vi "deviceAnalysisTest_DigitalTach.vi"() -> ()   [LabVIEW 2017]
uses:
  <vilib>/addons/InsightCM/MessageBus/Base/KeyValuePairs.ctl
  <vilib>/addons/InsightCM/MessageBus/Base/controls/AlarmRuleEntry.ctl
  <vilib>/addons/InsightCM/Devices/Shared/DataAccessors/controls/channelType_StatusLookup.ctl
  <vilib>/addons/InsightCM/MessageBus/Base/ConfigurableMetric.ctl
  <vilib>/addons/InsightCM/Utilities/ChannelStatus/controls/status.ctl
  <vilib>/addons/InsightCM/Utilities/ChannelStatus/controls/statusState.ctl
  <vilib>/addons/InsightCM/Devices/Shared/ConfigurationParsing/controls/filePaths.ctl
panel:
  out "seconds":i32
  out "logical OR":bool
  in  "Tachometer":cluster{"RPM":sgl}={"RPM"=60.0} {"RPM" scale=1.0..6000.0}
  in  "milliseconds to wait":u32=100
  in  "Tab Control":T1(tab)
  in  "Root Directory":path=path "C:/Users/Administrator/Desktop/testDevice files/speedProfile"
  in  "Configuration Files":T2={"AlarmRules"=path "AlarmRules.json", "MetricCfg"=path "MetricConfigs.json", "HierarchyNode"=path "Hierarchy.json", "DeviceModel"=path "DeviceModel.json"}
  in  "sampling info":cluster{"Fs":dbl, "#s":dbl}={"Fs"=10000.0, "#s"=10000.0} {"Fs" format="%.2p"}
  in  "Vibration":T3(array[cluster])
  out "Waveform Graph":waveform(dbl)[](graph)
  out "Waveform Graph 2":waveform(sgl)[](graph)
  out "FeatureLookup":variant
  in  "stop":bool
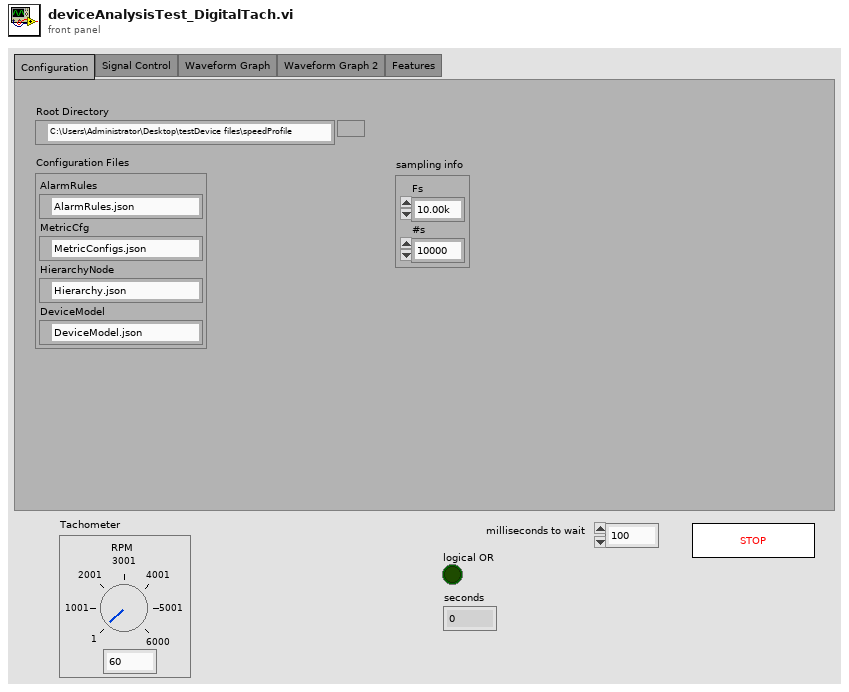
[diagram p1: front panel]
types:
  T1 = enum32{"Configuration", "Signal Control", "Waveform Graph", "Waveform Graph 2", "Features"}
  T2 = typedef "ConfigurationParsing.lvlib/filePaths.ctl" = cluster{"AlarmRules":path, "MetricCfg":path, "HierarchyNode":path, "DeviceModel":path}
  T3 = cluster{"order.":dbl, "mag (rms)":dbl, "phase (°)":dbl}[][]
  T4 = typedef "ChannelStatus.lvlib/statusState.ctl" = cluster{"channelAlias":string, "current":T5, "previous":T5, "changed":bool}
  T5 = typedef "ChannelStatus.lvlib/status.ctl" = enum16{"init", "ok", "open", "short", "outOfRange"}
  T6 = typedef "ConfigurableMetric.ctl" = cluster{"Id":i32, "MetricType":string, "Name":string, "Locked":bool, "Properties":T7}
  T7 = typedef "KeyValuePairs.ctl" = cluster{"Key":string, "Value":string}[]
  T8 = cluster{"order.":dbl, "mag (rms)":dbl, "phase (°)":dbl}[]
  T9 = typedef "AlarmRuleEntry.ctl" = cluster{"Id":i32, "State":string, "Path":string, "Message":string, "DeviceOnly":bool, "Configuration":cluster{"Condition":string, "SetPoint":string, "Type":string, "Hysteresis":dbl, "OnDelaySeconds":dbl, "OffDelaySeconds":dbl}, "Severity":i32}
  T10 = typedef "ConfigurationParsing.lvlib/DeviceConfigData.ctl" = cluster{"Device Info":T11, "AcquisitionProperties":variant, "Channels":variant[], "StreamingProperties":variant, "DeviceSystemProperties":variant}
  T11 = typedef "ConfigurationParsing.lvlib/deviceInfo.ctl" = cluster{"Config Version":string, "DeviceID":string}
  T12 = typedef "DeviceModel.ctl" = cluster{"AssetModel":T13, "SoftwareModel":T14}
  T13 = typedef "AssetModel.ctl" = cluster{"Id":i32, "PhysicalName":string, "LogicalName":string, "PluginCodename":string, "FirmwareInfo":string, "HardwareConfig":string, "SoftwareConfigId":i32, "HierarchyNodeId":i32}
  T14 = typedef "SoftwareModel.ctl" = cluster{"Id":i32, "DeviceAssetModelId":i32, "Version":string, "Config":string, "DeviceProperties":T7, "Channels":T15[]}
  T15 = typedef "BlueRidgeChannel.ctl" = cluster{"Id":i32, "ChannelId":string, "Name":string, "ChannelCategory":string, "ChannelType":string, "ChannelTypeList":string, "HierarchyNodeId":i32, "Enabled":bool, "Properties":T7, "MetricConfigurations":T16[]}
  T16 = typedef "MetricConfiguration.ctl" = cluster{"Id":i32, "ChannelCategory":string, "MeasurementType":string, "Metrics":T17[]}
  T17 = typedef "MetricInstance.ctl" = cluster{"Id":i32, "Codename":string, "DisplayName":string, "Unit":string, "Unscaled":bool, "Locked":bool, "TagPath":string, "Properties":T7}
  T18 = cluster{"AlarmRules":variant, "MetricCfg":variant, "HierarchyNode":variant, "DeviceConfig":T10, "DeviceModel":T12}
  T19 = typedef "AnalysisDevice.ctl" = cluster{"Device Id":string, "Dynamic Channels":T20[], "Static Channels":T28[]}
  T20 = typedef "AnalysisDynamicChannel.ctl" = cluster{"ChannelName":string, "Sensor Type":T21, "Conversion Op":T22, "Features":T23[], "Data":waveform(sgl), "Speed":sgl, "SP Index":i32, "Properties":variant, "Data Valid":bool, "Calc Measurement Type":T27}
  T21 = typedef "AnalysisSensorType.ctl" = enum16{"Accelerometer", "Velocity", "Displacement", "Tachometer", "Tempertature ", "dynamicVoltage", "Voltage", "Current", "Microphone", "Resistance", "Digital Input", "<Unknown>"}
  T22 = typedef "AnalysisConversionOp.ctl" = enum16{"none", "singleInt", "doubleInt", "singleDiff", "doubleDiff"}
  T23 = typedef "AnalysisFeature.ctl" = cluster{"Type":i32, "Code Name":string, "Unit":string, "Display Name":string, "Value":sgl, "Start":dbl, "Stop":dbl, "Band Domain":T24, "Band Calc":T25, "Amplitude Scale":T26, "Tag Path":string, "Conversion Op (phase sb only)":T22, "sbp code letter":string}
  T24 = typedef "AnalysisBandDomain.ctl" = enum16{"Frequency", "CPM", "Orders"}
  T25 = typedef "AnalysisBandCalculation.ctl" = enum16{"Total", "Max", "Phase"}
  T26 = typedef "AnalysisBandAmplitudeScale.ctl" = enum16{"rms", "peak", "pk-pk", "phase", "<none>"}
  T27 = typedef "AnalysisCalculatedMeasurementType.ctl" = enum16{"acceleration", "velocity", "displacement", "tachometer", "speed", "temperature", "voltage", "current", "resistance", "digitalInput", "<Unknown>"}
  T28 = typedef "AnalysisStaticChannel.ctl" = cluster{"ChannelName":string, "Sensor Type":T21, "Features":T23[], "Properties":variant, "Data Valid":bool, "Calc Measurement Type":T27, "Acquisition Timestamp":timestamp}
  T29 = typedef "AnalysisState.ctl" = cluster{"Properties":cluster{"File Properties":variant, "Static Properties":variant, "Waveform Properties":variant}, "Properties Initialized?":bool, "Device":T19, "Speed Profiles":T30[]}
  T30 = typedef "AnalysisSpeedProfile.ctl" = cluster{"t0":dbl, "pulse positions":sgl[], "speed":dbl}
  T31 = typedef "AnalysisBOP.lvlib/AnalysisGroups.ctl" = cluster{"StaticChannels":T32[], "TachVibrationGroups":T34[]}
  T32 = typedef "AnalysisBOP.lvlib/GeneralStaticChanAnalysisCfg.ctl" = cluster{"Wfm Index":i32, "ChannelName":string, "ChannelID":string, "bounds":T33, "TagPath":string, "Triggerable":bool}
  T33 = typedef "ChannelStatus.lvlib/outOfRangeBounds.ctl" = cluster{"maximum":dbl, "minimum":dbl}
  T34 = typedef "AnalysisBOP.lvlib/TachVibrationGroupCfg.ctl" = cluster{"TachometerChanAnalysisConfig":T35, "AnalysisChannels":T36[]}
  T35 = typedef "AnalysisBOP.lvlib/TachometerChanAnalysisCfg.ctl" = cluster{"Wfm Index":i32, "ChannelName":string, "ChannelID":string, "PulsesPerRevolution":sgl, "TachometerThreshold":sgl, "TachometerSlope":string, "TachometerHysteresis":sgl, "sampleRate":dbl, "tachometerType":string, "Analysis Wfm Index":i32}
  T36 = typedef "AnalysisBOP.lvlib/VibrationChanAnalysisCfg.ctl" = cluster{"Wfm Index":i32, "ChannelName":string, "ChannelID":string, "speedRatio":dbl, "MeasurementType":string}
  T37 = typedef "channelType_StatusLookup.ctl" = enum16{"Static", "Dynamic"}
  T38 = typedef "rolloverState.ctl" = cluster{"prev value":u32, "total add":dbl}
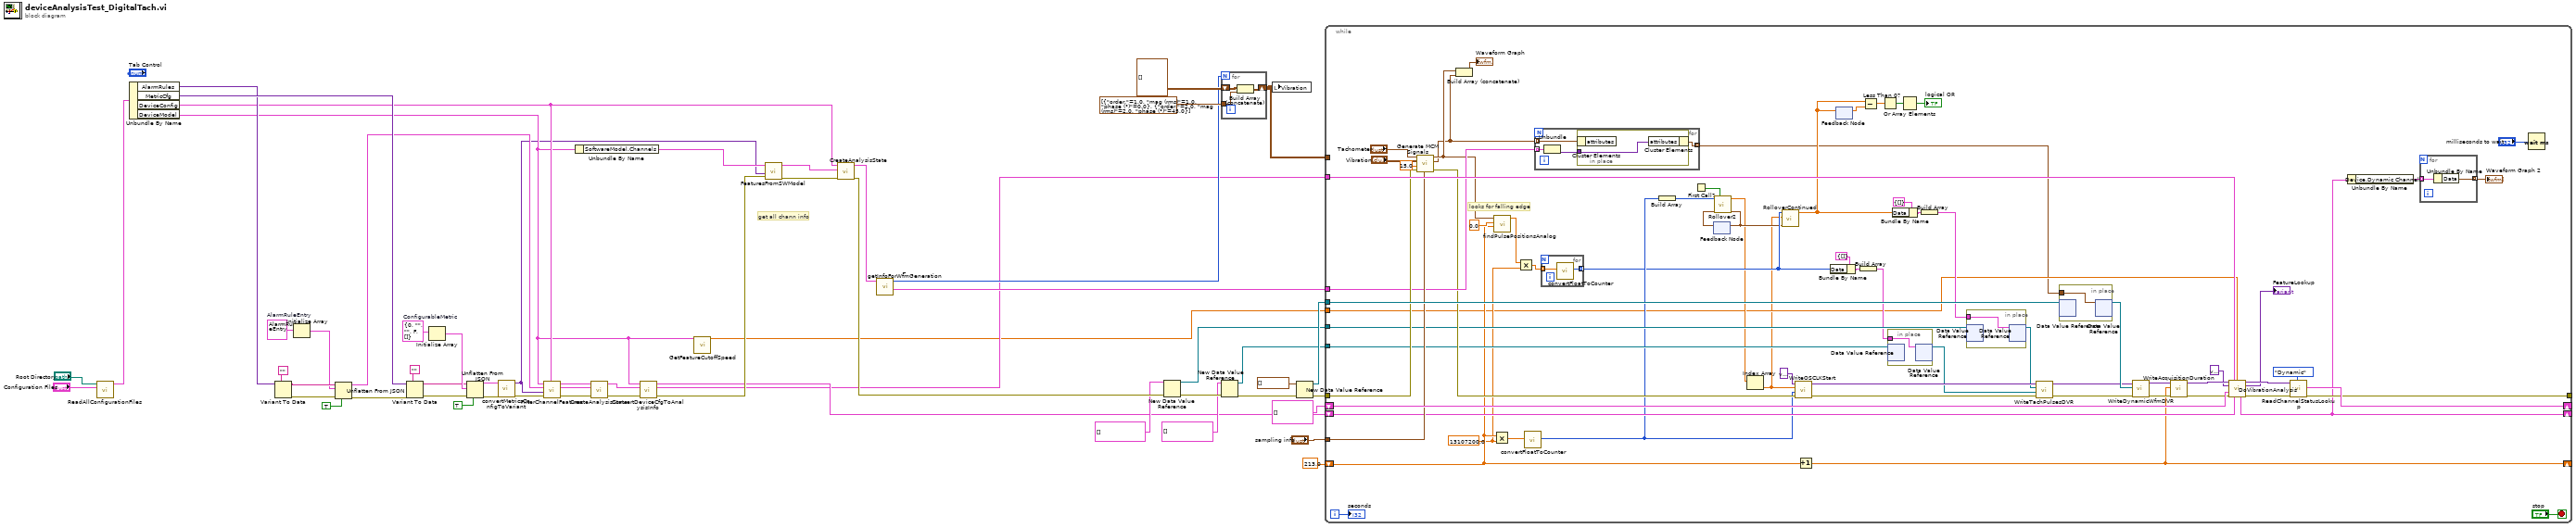
[diagram p0: block diagram]
diagram:
  w12 = T6 {"Id"=0, "MetricType"="", "Name"="", "Locked"=FALSE, "Properties"=[]}  # ConfigurableMetric
  w40 = T9 {"Id"=0, "State"="", "Path"="", "Message"="", "DeviceOnly"=FALSE, "Configuration"={"Condition"="", "SetPoint"="", "Type"="", "Hysteresis"=0.0, "OnDelaySeconds"=0.0, "OffDelaySeconds"=0.0}, "Severity"=0}  # AlarmRuleEntry
  # "get all chann info"
  n1 = call <vilib>:"ReadAllConfigurationFiles.vi"("Configuration Files"="Configuration Files", "Root Directory"="Root Directory") -> ("Configuration"=w52:T18)  [unwired: 6 in, 3 out]
  n2 = Unbundle By Name(w52) -> ("AlarmRules"=w37:variant, "MetricCfg"=w46:variant, "DeviceConfig"=w22:T10, "DeviceModel"=w5:T12)
  n3 = Variant To Data(type="", Variant=w37) -> (data=w41:string, error out=w43:errorcluster)  [unwired: 1 in]
  n4 = Initialize Array(w40) -> (w39:T9[])  [unwired: 1 in]
  n5 = Unflatten From JSON(JSON string=w41, type and defaults=w39, default null elements? (F)=TRUE, error in (no error)=w43) -> (value=w23:T9[], error out=w38:errorcluster)  [unwired: 3 in]
  n6 = Variant To Data(error in=w38, type="", Variant=w46) -> (data=w47:string, error out=w50:errorcluster)
  n7 = Initialize Array(w12) -> (w48:T6[])  [unwired: 1 in]
  n8 = Unflatten From JSON(JSON string=w47, type and defaults=w48, default null elements? (F)=TRUE, error in (no error)=w50) -> (value=w45:T6[], error out=w36:errorcluster)  [unwired: 3 in]
  n9 = call <vilib>:"convertMetricsConfigToVariant.vi"("error in (no error)"=w36, "MetricInstanceConfigs"=w45) -> ("error out"=w53:errorcluster, "metricInstanceConfig"=w1:variant)  [unwired: 8 in]
  n10 = call <vilib>:"FilterChannelFeatures.vi"("DeviceConfig"=w22, "error in (no error)"=w53, "Metric Lookup"=w1, "AlarmRules"=w23, "DeviceModel"=w5) -> ("error out"=w56:errorcluster, "Device"=w54:T19, "DeviceConfig Out"=w55:T10)  [unwired: 3 in, 1 out]
  n11 = Unbundle By Name(w5) -> ("SoftwareModel.Channels"=w13:T15[])
  n12 = call <vilib>:"CreateAnalysisState.vi"("error in (no error)"=w56, "Device"=w54, "DeviceConfig"=w55) -> ("error out"=w11:errorcluster, "Analysis State"=w10:T29)  [unwired: 7 in]
  n13 = call <vilib>:"ConvertDeviceCfgToAnalysisInfo.vi"("error in (no error)"=w11, "Analysis State"=w10, "DeviceModel"=w5) -> ("error out"=w9:errorcluster, "AnalysisGroups"=w7:T31, "Analysis State out"=w8:T29)  [unwired: 5 in, 1 out]
  n14 = call <vilib>:"GetFeatureCutoffSpeed.vi"("DeviceModel"=w5) -> ("featureCutoffSpeed"=w4:dbl)  [unwired: 10 in]
  n15 = call <vilib>:"FeaturesFromSWModel.vi"("error in (no error)"=w9, "Band Cache"=w1, "Channels"=w13) -> ("error out"=w3:errorcluster, "Device"=w2:T19)  [unwired: 7 in]
  n16 = call <vilib>:"CreateAnalysisState.vi"("error in (no error)"=w3, "Device"=w2, "DeviceConfig"=w22) -> ("error out"=w19:errorcluster, "Analysis State"=w24:T29)  [unwired: 7 in]
  n17 = call <vilib>:"_getInfoForWfmGeneration.vi"("Analysis State"=w24) -> ("wfm info"=w25:cluster{i32, "variant":variant}[], "number of channels"=w26:i32)  [unwired: 9 in]
  n18 = New Data Value Reference(data value=cluster{"Data":dbl[]}[] [] ("Keyphasor Pulses"), error in=w19) -> (data value reference=w15:refnum<data-value>, error out=w20:errorcluster)
  n19 = New Data Value Reference(data value=cluster{"Data":u32[]}[] [] ("Keyphasor Pulses U32"), error in=w20) -> (data value reference=w16:refnum<data-value>, error out=w21:errorcluster)
  n20 = for {
    N: w26 -> [_]
    tunnel: T8 [{"order."=1.0, "mag (rms)"=1.0, "phase (°)"=0.0}, {"order."=2.0, "mag (rms)"=2.0, "phase (°)"=45.0}] ("Vibration") -> [w59]
    shift-right: [w58] -> w28
    shift-left: T3 [] -> [w57]
    n21 = Build Array (concatenate)(w57, w59) -> (w58:T3)
  }
  n22 = local write "Vibration"(w28) -> ()
  n23 = New Data Value Reference(data value=waveform(sgl)[] [] ("wfmData"), error in=w21) -> (data value reference=w32:refnum<data-value>, error out=w33:errorcluster)
  n24 = while {
    tunnel: w33 -> [w117]
    tunnel: w7 -> [w128]
    shift-right: [w127] -> _
    shift-left: T4[] [] ("channel status") -> [w126]
    tunnel: w32 -> [w121]
    tunnel: "sampling info" -> [w115]
    tunnel: w28 -> [_]
    tunnel: [w109] -> _
    tunnel: w25 -> [w108]
    shift-right: [w106] -> _
    shift-left: w8 -> [w107]
    tunnel: w16 -> [w96]
    tunnel: w15 -> [w97]
    shift-right: [w88] -> _
    shift-left: 213.0 -> [w87]
    tunnel: w4 -> [w72]
    i -> [w66]
    stop <- "stop" stop-if-true
    w85 = 13107200.0
    # "looks for falling edge"
    n25 = call <vilib>:"Generate MCM Signals.vi"("sampling info"=w115, "error in"=w117, "square wave duty cycle (%)"=15.0, "Vibration"="Vibration", "Tachometer"="Tachometer") -> ("error out"=w98:errorcluster, "Vibration signals"=w62:waveform(dbl)[], "Tach signal"=w63:waveform(dbl))  [unwired: 4 in]
    n26 = Build Array (concatenate)(w63, w62) -> (→"Waveform Graph":waveform(dbl)[])
    n27 = Multiply(x=w87, y=w85) -> (x*y=w80:dbl)
    n28 = call <vilib>:"findPulsePositionsAnalog.vi"("t0"=w87, "Level"=0.0, "Tach signal"=w63) -> ("pulse positions"=w86:dbl[])  [unwired: 8 in]
    n29 = Multiply(x=w86, y=w85) -> (x*y=w81:dbl[])
    n30 = call <vilib>:"convertFloatToCounter.vi"("Numeric"=w80) -> ("Counter Version"=w78:u32)  [unwired: 10 in]
    n31 = for {
      tunnel: w62 -> [w137] mode=indexing
      tunnel: w108 -> [w138] mode=indexing
      tunnel: [w136] -> w65 mode=indexing
      n32 = Unbundle(w138) -> ("variant"=w135:variant)  [unwired: 1 out]
      n33 = in-place {
        in-place-border: w135 -> [w139]
        n34 = in-place-cluster #1(w137) -> ()  [unwired: 1 out]
        n35 = in-place-cluster #1("attributes"=w139) -> (w136:waveform(dbl))
      }
    }
    n36 = for {
      tunnel: w81 -> [w130] mode=indexing
      tunnel: [w129] -> w75 mode=indexing
      n37 = call <vilib>:"convertFloatToCounter.vi"("Numeric"=w130) -> ("Counter Version"=w129:u32)  [unwired: 10 in]
    }
    n38 = Build Array(w78) -> (w76:u32[])
    n39 = First Call?() -> (First Call?: T/F=w79:bool)
    n40 = feedback #2() -> (w77:T38)  [unwired: 1 in]
    n41 = call <vilib>:"Rollover2.vi"("reset"=w79, "rollover state"=w77, "counter"=w76) -> ("rollover state"=w74:T38, "counter"=w73:dbl[])  [unwired: 7 in]
    n42 = feedback-in #2(w74) -> ()
    n43 = Index Array(array=w73) -> (element=w60:dbl)  [unwired: 1 in]
    n44 = call <vilib>:"RolloverContinued.vi"("rollover state"=w74, "OSClkStart"=w60, "counter"=w75) -> ("this block"=w71:dbl[])  [unwired: 5 in, 3 out]
    n45 = call <vilib>:"WriteOSCLKStart.vi"("error in (no error)"=w98, "osclkStart U32"=w78, "osclkStart"=w60, "variant"=variant) -> ("error out"=w101:errorcluster, "variant"=w102:variant)  [unwired: 6 in]
    n46 = Increment(x=w87) -> (x+1=w88:dbl)
    n47 = Bundle By Name(cluster=cluster{"Data":u32[]} {"Data"=[]} ("PulsePositions"), "Data"=w75) -> (w84:cluster{"Data":u32[]})
    n48 = feedback-in #3(w71) -> ()
    n49 = feedback #3() -> (w70:dbl[])  [unwired: 1 in]
    n50 = Build Array(w84) -> (w82:cluster{"Data":u32[]}[])
    n51 = Subtract(x=w71, y=w70) -> (x-y=w69:dbl[])
    n52 = Less Than 0?(x=w69) -> (x < 0?=w68:bool[])
    n53 = in-place {
      in-place-border: w82 -> [w131]
      n54 = in-place-dvr #4(w96) -> ()  [unwired: 2 out]
      n55 = in-place-dvr #4(w131) -> (w95:refnum<data-value>)  [unwired: 1 out]
    }
    n56 = Bundle By Name(cluster=cluster{"Data":dbl[]} {"Data"=[]} ("PulsePositions"), "Data"=w71) -> (w90:cluster{"Data":dbl[]})
    n57 = Or Array Elements(Boolean array=w68) -> (logical OR=→"logical OR":bool)
    n58 = Build Array(w90) -> (w89:cluster{"Data":dbl[]}[])
    n59 = in-place {
      in-place-border: w89 -> [w132]
      n60 = in-place-dvr #5(w97) -> ()  [unwired: 2 out]
      n61 = in-place-dvr #5(w132) -> (w94:refnum<data-value>)  [unwired: 1 out]
    }
    n62 = call <vilib>:"WriteTachPulsesDVR.vi"("error in (no error)"=w101, "tachometer pulses U32"=w95, "tachometerPulsesDVR"=w94, "variant"=w102) -> ("error out"=w100:errorcluster, "variant"=w93:variant)  [unwired: 6 in]
    n63 = in-place {
      in-place-border: w65 -> [w140]
      n64 = in-place-dvr #6(w121) -> ()  [unwired: 2 out]
      n65 = in-place-dvr #6(w140) -> (w120:refnum<data-value>)  [unwired: 1 out]
    }
    n66 = call <vilib>:"WriteDynamicWfmDVR.vi"("error in (no error)"=w100, "dynamic Wfm DVR"=w120, "variant"=w93) -> ("error out"=w125:errorcluster, "variant"=w124:variant)  [unwired: 7 in]
    n67 = call <vilib>:"WriteAcquisitionDuration.vi"("error in (no error)"=w125, "acquisitionDuration"=w88, "variant"=w124) -> ("error out"=w122:errorcluster, "variant"=w123:variant)  [unwired: 7 in]
    n68 = call <vilib>:"DoVibrationAnalysis.vi"("variant"=w123, "AnalysisGroups"=w128, "FeatureSpeedCutoff"=w72, "featureLookup"=variant, "channel status"=w126, "error in (no error)"=w122, "Analysis State"=w107) -> ("variant out"=w112:variant, "FeatureLookup"=→"FeatureLookup":variant, "Analysis State Out"=w106:T29, "error out"=w111:errorcluster)  [unwired: 4 in, 1 out]
    n69 = call <vilib>:"ReadChannelStatusLookup.vi"("channel type"=channelType_StatusLookup."Dynamic", "error in (no error)"=w111, "variant"=w112) -> ("error out"=w109:errorcluster, "channel status"=w127:T4[])  [unwired: 6 in, 1 out]
    n70 = Unbundle By Name(w106) -> ("Device.Dynamic Channels"=w105:T20[])
    n71 = for {
      tunnel: w105 -> [w134] mode=indexing
      tunnel: [w133] -> w104 mode=indexing
      n72 = Unbundle By Name(w134) -> ("Data"=w133:waveform(sgl))
    }
    "Waveform Graph 2" <- w104
    n73 = Wait (ms)(milliseconds to wait="milliseconds to wait") -> ()  [unwired: 1 out]
    "seconds" <- w66
  }
